vi "lowerBoundOnTable.vi"(4 "column_to_sort":i32, 5 "sign":dbl, 6 "sign_idx":i32, 7 "table":dbl[][](array[numeric]), 8 "error in (no error)":errorcluster, 9 "target_idx":i32, 10 "key":dbl, 11 "Game in":refnum<class "Game.lvclass">) -> (0 "error out":errorcluster, 2 "search_results":dbl[][](array[numeric]), 3 "Game out":refnum<class "Game.lvclass">)   [LabVIEW 2021, in "Game.lvclass"]
uses:
  Game.lvclass
  1b529bbd-c979-4235-975a-70d1ab09a3d3.vi
  <vilib>/Array/Sort 2D Array - Pop Stack.vi
  <vilib>/Array/Sort 2D Array - Push Stack.vi
  1b529bbd-c979-4235-975a-70d1ab09a3d3.vi/269d4b3b-47f5-49e3-8884-44851e4dd9d5.vi
  1b529bbd-c979-4235-975a-70d1ab09a3d3.vi/6d99389c-673d-4efb-bf33-19b32bcf4cf8.vi
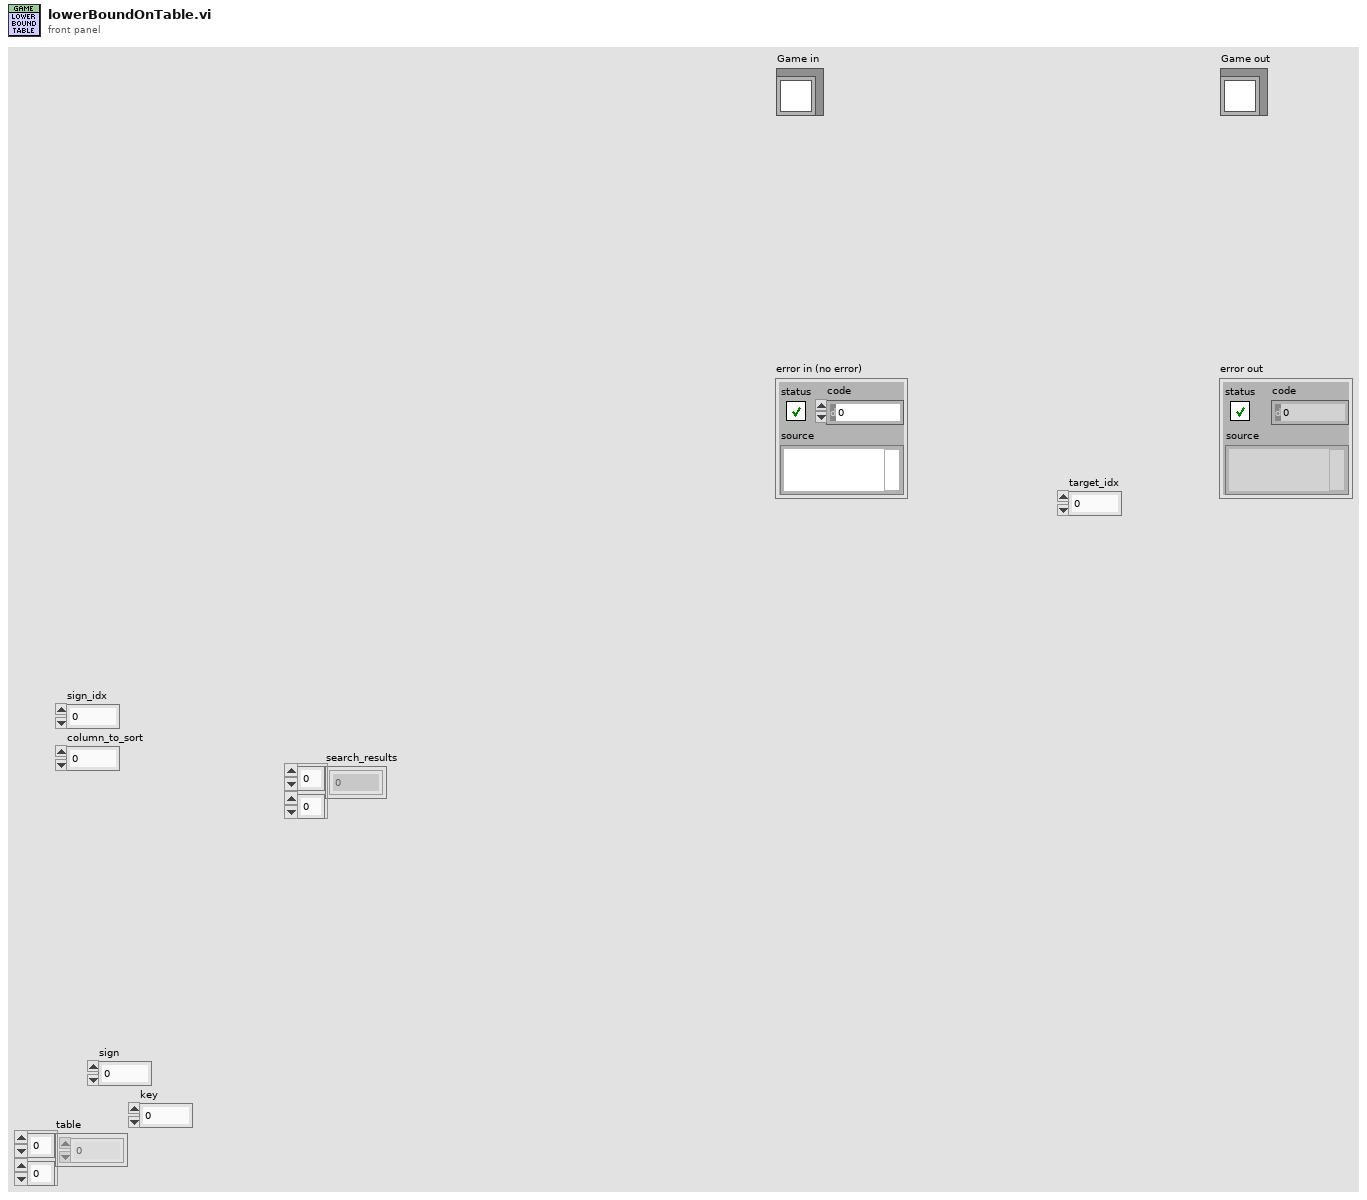
[diagram p1: front panel]
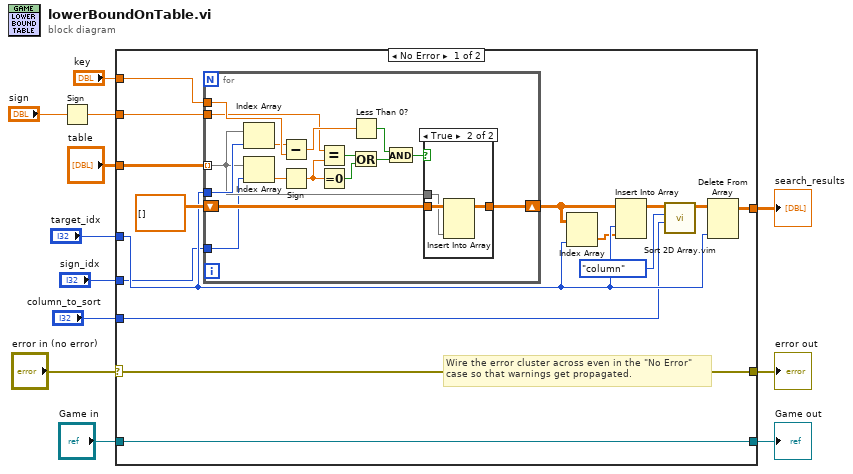
[diagram p0: block diagram]
diagram:
  n1 = Sign(1:"sign") -> (0:w3:dbl)
  n2 = case shown="No Error" "error in (no error)" {
    selector: "error in (no error)" -> [w26 w49]
    tunnel: [w26 w49] -> w11
    tunnel: [w27 w48] -> w9
    tunnel: "Game in" -> [w27 w48]
    tunnel: "key" -> [w20 _]
    tunnel: "table" -> [w19 _]
    tunnel: w3 -> [w16 _]
    tunnel: "target_idx" -> [w18 _]
    tunnel: [w17 _] -> w5
    tunnel: "sign_idx" -> [w14 _]
    tunnel: "column_to_sort" -> [w13 _]
    frame No Error {
      # "Wire the error cluster across even in the \"No Error\"\ncase so that warnings get propagated."
      n3 = for {
        tunnel: w19 -> [w37] mode=indexing
        tunnel: w20 -> [w43]
        shift-right: [w41] -> w23
        shift-left: dbl[][] [] ("appended array") -> [w42]
        tunnel: w18 -> [w39]
        tunnel: w16 -> [w33]
        tunnel: w14 -> [w36]
        n4 = Index Array(array=w37, index=w39) -> (element=w40:dbl)
        n5 = Index Array(array=w37, index=w36) -> (element=w35:dbl)
        n6 = Subtract(x=w40, y=w43) -> (x-y=w38:dbl)
        n7 = Sign(1:w35) -> (0:w32:dbl)
        n8 = Equal?(x=w33, y=w32) -> (x = y?=w31:bool)
        n9 = Equal To 0?(x=w32) -> (x = 0?=w34:bool)
        n10 = Less Than 0?(x=w38) -> (x < 0?=w30:bool)
        n11 = Or(x=w31, y=w34) -> (x .or. y?=w29:bool)
        n12 = And(x=w30, y=w29) -> (x .and. y?=w28:bool)
        n13 = case shown="True" w28 {
          tunnel: w42 -> [w44 w47]
          tunnel: w37 -> [_ w46]
          tunnel: [w44 w45] -> w41
          frame False {
          }
          frame True {
            n14 = Insert Into Array(array=w47, new element=w46) -> (w45:dbl[][])  [unwired: 2 in]
          }
        }
      }
      n15 = Index Array(array=w23, index (col)=w18) -> (element=w15:dbl[])  [unwired: 1 in]
      n16 = Insert Into Array(array=w23, index (col)=w18, new element=w15) -> (w22:dbl[][])  [unwired: 1 in]
      n17 = call "Sort 2D Array.vim"("index"=w13, "dimension to index (column)"=enum16{"column", "row"}."column", "2D array"=w22) -> ("sorted 2D array"=w21:dbl[][])  [unwired: 7 in, 1 out]
      n18 = Delete From Array(array=w21, index (col)=w18) -> (array with subset deleted=w17:dbl[][])  [unwired: 2 in, 1 out]
    }
    frame Error {
    }
  }
  "error out" <- w11
  "Game out" <- w9
  "search_results" <- w5
